vi "TxPkt - Export Channel Configuration.vi"(8 "error in (no error)":errorcluster, 11 "Packet Ref in":T1 format="%.0x") -> (0 "error out":errorcluster, 3 "Packet Ref out":T1 format="%.0x")   [LabVIEW 2016, in "UDP-Custom-Device System Explorer.lvlib"]
uses:
  UDP-Custom-Device System Explorer.lvlib
  <vilib>/NI Veristand/Custom Device API/Custom Device Item Ref.ctl
  Types/Channel Configuration/Channel Config File Data.ctl
  Property Accessors/Tx Packet Accessors.lvlib
  Property Accessors/Shared Packet Accessors.lvlib
  <vilib>/NI VeriStand/Custom Device API/Custom Device API.lvlib
  Shared/UDP-Custom-Device Shared.lvlib
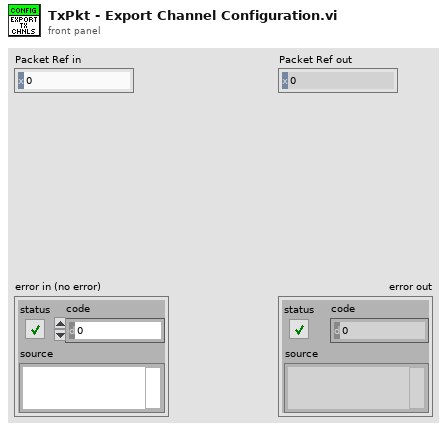
[diagram p1: front panel]
types:
  T1 = typedef "Custom Device API.lvlib/Custom Device Item Ref.ctl" = u64
  T2 = typedef "Channel Config File Data.ctl" = cluster{"Signal Names":string[], "Channel Names":string[], "Channel Data Types":string[], "Channel Descriptions":string[]}
  T3 = typedef "UDP-Custom-Device Shared.lvlib/Shared - Channel Data Type.ctl" = enum16{"Boolean", "Single", "Double", "I8", "I16", "I32", "I64", "U8", "U16", "U32", "U64"}
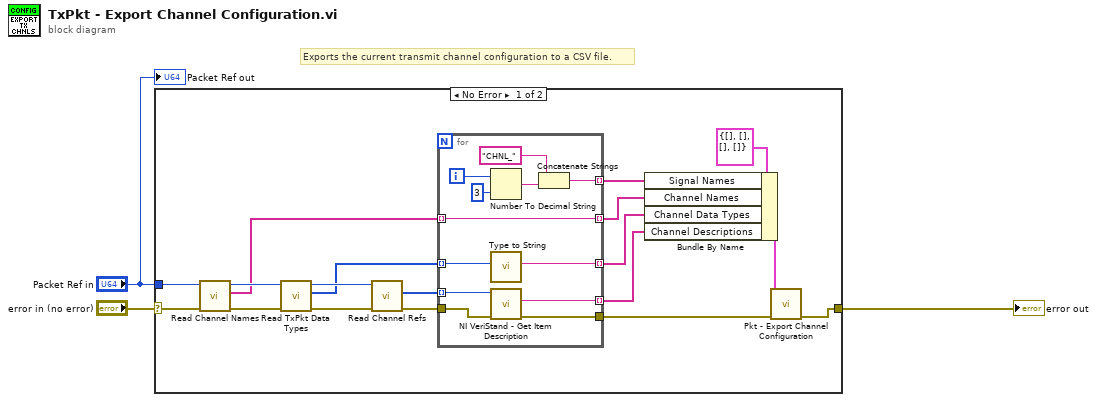
[diagram p0: block diagram]
diagram:
  # "Exports the current transmit channel configuration to a CSV file."
  n1 = case shown="No Error" "error in (no error)" {
    selector: "error in (no error)" -> [w20 w34]
    tunnel: "Packet Ref in" -> [w21 _]
    tunnel: [w10 w34] -> w2
    frame No Error {
      n2 = call "Read Channel Names.vi"("error in (no error)"=w20, "Node Ptr"=w21) -> ("error out"=w18:errorcluster, "Channel Names"=w12:string[], "Node Ptr out"=w19:T1)  [unwired: 7 in]
      n3 = call "Read TxPkt Data Types.vi"("error in (no error)"=w18, "Node Ptr"=w19) -> ("error out"=w16:errorcluster, "Data types"=w13:T3[], "Node Ptr out"=w17:T1)  [unwired: 7 in]
      n4 = call "Read Channel Refs.vi"("error in (no error)"=w16, "Node Ptr"=w17) -> ("error out"=w15:errorcluster, "Dependent Node Refs"=w14:T1[])  [unwired: 7 in, 1 out]
      n5 = for {
        tunnel: w15 -> [w32]
        tunnel: w14 -> [w33] mode=indexing
        tunnel: [w31] -> w5 mode=indexing
        tunnel: [w30] -> w11
        tunnel: w13 -> [w25] mode=indexing
        tunnel: [w24] -> w6 mode=indexing
        tunnel: [w23] -> w8 mode=indexing
        tunnel: w12 -> [w22] mode=indexing
        tunnel: [w22] -> w7 mode=indexing
        i -> [w28]
        n6 = Number To Decimal String(number=w28, width (-)=i16 3) -> (decimal integer string=w26:string)
        n7 = call "Type to String.vi"("Data Type"=w25) -> ("String Type"=w24:string)  [unwired: 10 in]
        n8 = call <vilib>:"NI VeriStand - Get Item Description.vi"("error in (no error)"=w32, "Item Ref in"=w33) -> ("error out"=w30:errorcluster, "Description"=w31:string)  [unwired: 6 in, 2 out]
        n9 = Concatenate Strings("CHNL_" ("Description"), w26) -> (w23:string)
      }
      n10 = Bundle By Name(cluster=T2 {"Signal Names"=[], "Channel Names"=[], "Channel Data Types"=[], "Channel Descriptions"=[]} ("Channel Config Data"), "Signal Names"=w8, "Channel Names"=w7, "Channel Data Types"=w6, "Channel Descriptions"=w5) -> (w4:T2)
      n11 = call "Pkt - Export Channel Configuration.vi"("error in (no error)"=w11, "Channel Config Data"=w4) -> ("error out"=w10:errorcluster)  [unwired: 9 in]
    }
    frame Error {
    }
  }
  "error out" <- w2
  "Packet Ref out" <- "Packet Ref in"
